vi "2D array sort with key_column.vi"(1 "ascending":bool, 2 "key column":u16, 3 "input":dbl[][](array[numeric])) -> (0 "output":dbl[][](array[numeric]))   [LabVIEW 2019]
panel:
  out "size(s)":i32[](array[numeric])
  # "descending"
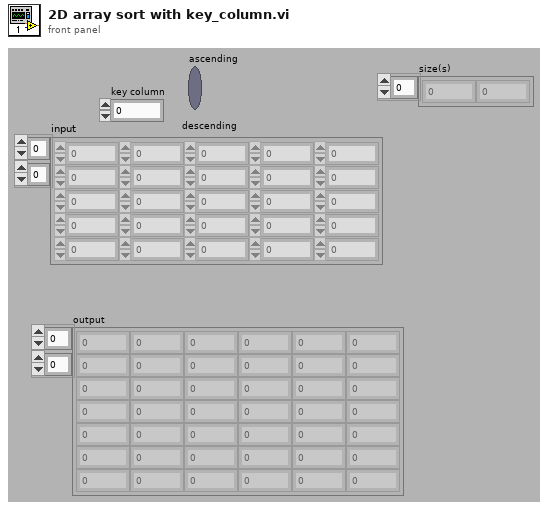
[diagram p1: front panel]
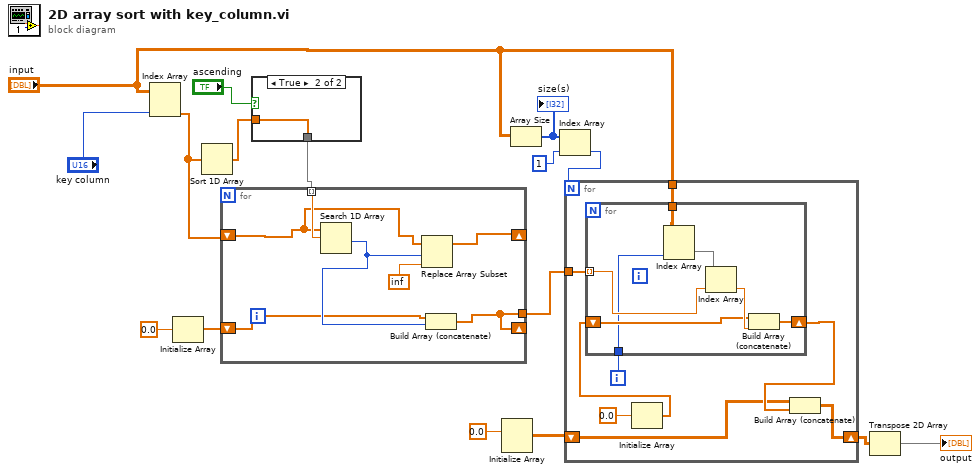
[diagram p0: block diagram]
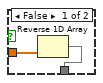
[diagram p2: hidden frame]
diagram:
  n1 = Index Array(array="input", index (col)="key column") -> (element=w13:dbl[])  [unwired: 1 in]
  n2 = Initialize Array(0.0 ("element")) -> (w14:dbl[])  [unwired: 1 out]
  n3 = Sort 1D Array(array=w13) -> (sorted array=w6:dbl[])
  n4 = case shown="True" "ascending" {
    tunnel: [w17 w19] -> w7
    tunnel: w6 -> [w18 w19]
    frame False {
      n5 = Reverse 1D Array(array=w18) -> (reversed array=w17:dbl[])
    }
    frame True {
    }
  }
  n6 = for {
    tunnel: w7 -> [w26] mode=indexing
    tunnel: [w22] -> w16
    shift-right: [w23] -> _
    shift-left: w13 -> [w24]
    shift-right: [w22] -> _
    shift-left: w14 -> [w21]
    n7 = Search 1D Array(1D array=w24, element=w26) -> (index of element=w25:i32)  [unwired: 1 out]
    n8 = Replace Array Subset(array=w24, new element=inf, index=w25) -> (w23:dbl[])
    n9 = Build Array (concatenate)(w21, w25) -> (w22:dbl[])
  }
  n10 = Initialize Array(0.0 ("element")) -> (w8:dbl[][])  [unwired: 2 out]
  n11 = Array Size(array="input") -> (size(s)=w12:i32[])
  "size(s)" <- w12
  n12 = Index Array(array=w12, index=1) -> (element=w10:i32)
  n13 = for {
    N: w10 -> [_]
    tunnel: w16 -> [w34]
    tunnel: "input" -> [w33]
    shift-right: [w27] -> w3
    shift-left: w8 -> [w28]
    i -> [w32]
    n14 = Initialize Array(0.0 ("element")) -> (w30:dbl[])  [unwired: 1 out]
    n15 = for {
      shift-right: [w36] -> w29
      shift-left: w30 -> [w37]
      tunnel: w34 -> [w39] mode=indexing
      tunnel: w33 -> [w41]
      tunnel: w32 -> [w35]
      n16 = Index Array(array=w41, index (col)=w35) -> (element=w40:dbl[])  [unwired: 1 in]
      n17 = Index Array(array=w40, index=w39) -> (element=w38:dbl)
      n18 = Build Array (concatenate)(w37, w38) -> (w36:dbl[])
    }
    n19 = Build Array (concatenate)(w28, w29) -> (w27:dbl[][])
  }
  n20 = Transpose 2D Array(2D array=w3) -> (transposed array=→"output":dbl[][])
